vi "Simulate RC Arm.vi"   [LabVIEW 2014]
types:
  T1 = cluster{"chan1_raw":u16, "chan2_raw":u16, "chan3_raw":u16, "chan4_raw":u16, "chan5_raw":u16, "chan6_raw":u16, "chan7_raw":u16, "chan8_raw":u16, "target_system":u8, "target_component":u8}
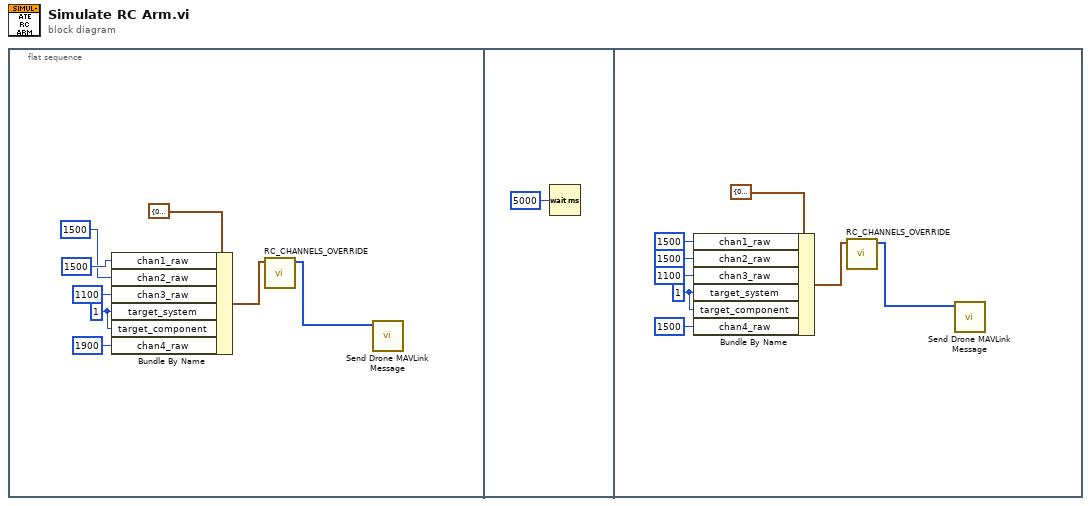
[diagram p0: block diagram]
diagram:
  n1 = flat-sequence {
    frame #0 {
      w7 = u8 1 ("target_system")
      n2 = Bundle By Name(cluster=T1 {"chan1_raw"=0, "chan2_raw"=0, "chan3_raw"=0, "chan4_raw"=0, "chan5_raw"=0, "chan6_raw"=0, "chan7_raw"=0, "chan8_raw"=0, "target_system"=0, "target_component"=0} ("Payload"), "chan1_raw"=u16 1500 ("chan2_raw"), "chan2_raw"=u16 1500 ("chan1_raw"), "chan3_raw"=u16 1100, "target_system"=w7, "target_component"=w7, "chan4_raw"=u16 1900) -> (w5:T1)
      n3 = call "RC_CHANNELS_OVERRIDE.vi"("Payload"=w5) -> ("MAVLink Message"=w4:u8[])  [unwired: 10 in]
      n4 = call "Send Drone MAVLink Message.vi"("MAVLink Message"=w4) -> ()  [unwired: 10 in, 1 out]
    }
    frame #1 {
      n5 = Wait (ms)(milliseconds to wait=u32 5000) -> ()  [unwired: 1 out]
    }
    frame #2 {
      w12 = u8 1 ("target_system")
      n6 = Bundle By Name(cluster=T1 {"chan1_raw"=0, "chan2_raw"=0, "chan3_raw"=0, "chan4_raw"=0, "chan5_raw"=0, "chan6_raw"=0, "chan7_raw"=0, "chan8_raw"=0, "target_system"=0, "target_component"=0} ("Payload"), "chan1_raw"=u16 1500, "chan2_raw"=u16 1500, "chan3_raw"=u16 1100, "target_system"=w12, "target_component"=w12, "chan4_raw"=u16 1500) -> (w16:T1)
      n7 = call "RC_CHANNELS_OVERRIDE.vi"("Payload"=w16) -> ("MAVLink Message"=w17:u8[])  [unwired: 10 in]
      n8 = call "Send Drone MAVLink Message.vi"("MAVLink Message"=w17) -> ()  [unwired: 10 in, 1 out]
    }
  }
